vi "DAQ comm.vi"(7 "DAQ T state cluster in":T1={"DAQ state"=enum."Global comm", "device"="Dev1", "start (ms)"=0, "error"={"status"=FALSE, "code"=0, "source"=""}, "T cont"={"exec"={"T mode"=enum."Setting up", "man power"=0.0, "log"=FALSE}, "T status"={"Temp"=0.0, "Power"=0.0}, "utility"={"meas index"=300, "wait (ms)"=0, "H Vmax"=8.5, "power out"=0.0, "heat volt out"=0.0, "heat volt in"=0.0, "therm volt"=0.0, "t T P hist"=[]}}} {"T cont"."utility"."therm volt" format="%_6g"; "T cont"."utility"."heat volt in" format="%_6g"; "T cont"."utility"."heat volt out" format="%_6g"; "T cont"."utility"."power out" format="%_6g"; "T cont"."utility"."H Vmax" format="%_6g"; "T cont"."exec"."man power" format="%_6g"; "T cont"."T status"."Power" format="%_6g"; "T cont"."T status"."Temp" format="%_6g"}) -> (8 "DAQ T state cluster out":T1={"DAQ state"=enum."Global comm", "device"="Dev1", "start (ms)"=0, "error"={"status"=FALSE, "code"=0, "source"=""}, "T cont"={"exec"={"T mode"=enum."Listening to exec", "man power"=0.0, "log"=FALSE}, "T status"={"Temp"=0.0, "Power"=0.0}, "utility"={"meas index"=0, "wait (ms)"=0, "H Vmax"=8.5, "power out"=5.0, "heat volt out"=0.0, "heat volt in"=0.0, "therm volt"=0.0, "t T P hist"=[]}}} {"T cont"."utility"."therm volt" format="%_6g"; "T cont"."utility"."heat volt in" format="%_6g"; "T cont"."utility"."heat volt out" format="%_6g"; "T cont"."utility"."power out" format="%_6g"; "T cont"."utility"."H Vmax" format="%_6g"; "T cont"."exec"."man power" format="%_6g"; "T cont"."T status"."Power" format="%_6g"; "T cont"."T status"."Temp" format="%_6g"})   [LabVIEW 2019]
doc: "This subVI is one of the states of the DAQ state machine in the bug experiment.\n\nThis state monitors the global variables used in the bug experiment. Depending upon the T control mode, it can be transient, or a dwell state with indefinite dwell time while waiting to engage the DAQ interfacing.\n\nPaul K Dixon\nP3600\nCSUSB Physics"
uses:
  typedefs/DAQ T state cluster.ctl
  typedefs/DAQ T state enum.ctl
  typedefs/temp cont cluster.ctl
  typedefs/temp exec cluster.ctl
  typedefs/temp mode enum.ctl
  typedefs/temp indicator.ctl
  typedefs/temp cont utility.ctl
  globals/Bug man temp globals.vi
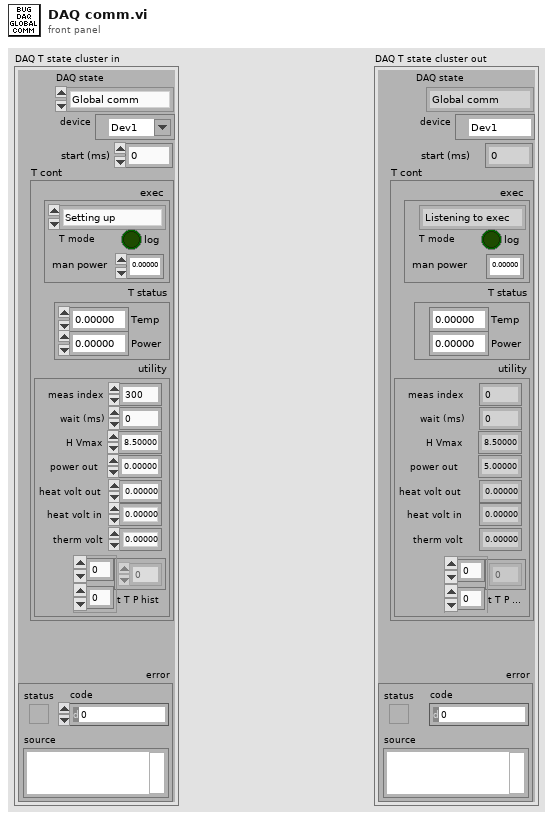
[diagram p1: front panel]
types:
  T1 = typedef "DAQ T state cluster.ctl" = cluster{"DAQ state":T2, "device":tag, "start (ms)":i32, "error":errorcluster, "T cont":T3}
  T2 = typedef "DAQ T state enum.ctl" = enum16{"Global comm", "Meas T & P", "Man Power set", "Output Power", "Wait", "Exit"}
  T3 = typedef "temp cont cluster.ctl" = cluster{"exec":T4, "T status":T6, "utility":T7}
  T4 = typedef "temp exec cluster.ctl" = cluster{"T mode":T5, "man power":dbl, "log":bool}
  T5 = typedef "temp mode enum.ctl" = enum16{"Setting up", "Listening to exec", "Exit"}
  T6 = typedef "temp indicator.ctl" = cluster{"Temp":dbl, "Power":dbl}
  T7 = typedef "temp cont utility.ctl" = cluster{"meas index":i32, "wait (ms)":i32, "H Vmax":dbl, "power out":dbl, "heat volt out":dbl, "heat volt in":dbl, "therm volt":dbl, "t T P hist":dbl[][]}
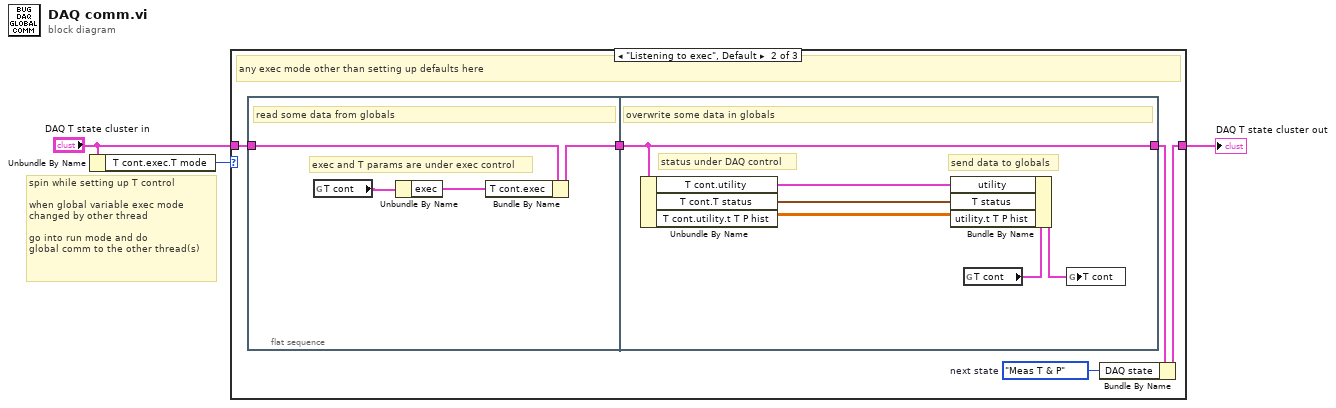
[diagram p0: block diagram]
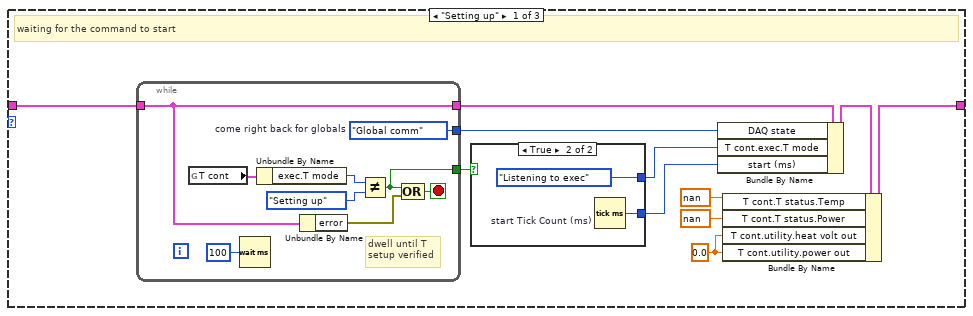
[diagram p2: hidden frame]
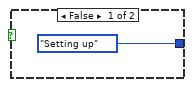
[diagram p3: hidden frame]
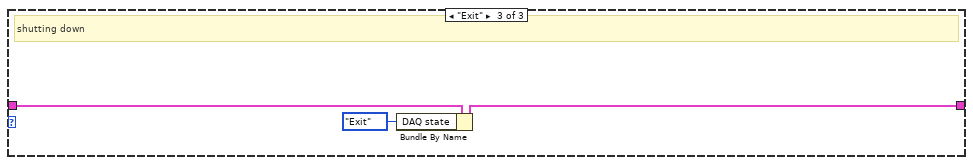
[diagram p4: hidden frame]
diagram:
  # "spin while setting up T control \n\nwhen global variable exec mode\nchanged by other thread\n\ngo into run mode and do\nglobal comm to the other thread(s)"
  n1 = Unbundle By Name("DAQ T state cluster in") -> ("T cont.exec.T mode"=w3:T5)
  n2 = case shown="\"Listening to exec\", Default" w3 {
    tunnel: "DAQ T state cluster in" -> [w14 w31 w44]
    tunnel: [w7 w30 w43] -> w1
    frame "Setting up" {
      w4 = 0.0 ("T cont.heat volt out")
      # "waiting for the command to start"
      n3 = while {
        tunnel: w14 -> [w24]
        tunnel: [w24] -> w13
        tunnel: [w22] -> w12
        tunnel: [w18] -> w10
        stop <- w26 stop-if-true
        w22 = DAQ_T_state_enum."Global comm"  # come right back for globals
        # "dwell until T \nsetup verified"
        n4 = global read "Bug man temp globals.vi" "T cont"() -> (w21:T3)
        n5 = Wait (ms)(milliseconds to wait=u32 100) -> ()  [unwired: 1 out]
        n6 = Unbundle By Name(w21) -> ("exec.T mode"=w20:T5)
        n7 = Unbundle By Name(w24) -> ("error"=w25:errorcluster)
        n8 = Not Equal?(x=w20, y=temp_mode_enum."Setting up" ("exec.T mode")) -> (x != y?=w18:bool)
        n9 = Compound Arithmetic op=OR(w18, w25) -> (w26:bool)
      }
      n10 = case shown="True" w10 {
        tunnel: [temp_mode_enum."Setting up" ("T cont.exec.T mode") temp_mode_enum."Listening to exec" ("T cont.exec.T mode")] -> w11
        tunnel: [_ w16] -> w9
        frame False {
        }
        frame True {
          n11 = Tick Count (ms) "start Tick Count (ms)"() -> (millisecond timer value=w16:u32)
        }
      }
      n12 = Bundle By Name(cluster=w13, "DAQ state"=w12, "T cont.exec.T mode"=w11, "start (ms)"=w9) -> (w8:T1)
      n13 = Bundle By Name(cluster=w8, "T cont.T status.Temp"=nan, "T cont.T status.Power"=nan, "T cont.utility.heat volt out"=w4, "T cont.utility.power out"=w4) -> (w7:T1)
    }
    frame "Listening to exec", Default {
      w29 = DAQ_T_state_enum."Meas T & P"  # next state
      # "any exec mode other than setting up defaults here"
      n14 = flat-sequence {
        tunnel: w31 -> [w35]
        tunnel: [w32] -> w27
        tunnel: [w36] -> w28
        tunnel: w27 -> [w36]
        frame #0 {
          # "exec and T params are under exec control"
          # "read some data from globals"
          n15 = global read "Bug man temp globals.vi" "T cont"() -> (w34:T3)
          n16 = Unbundle By Name(w34) -> ("exec"=w33:T4)
          n17 = Bundle By Name(cluster=w35, "T cont.exec"=w33) -> (w32:T1)
        }
        frame #1 {
          # "status under DAQ control"
          # "send data to globals"
          # "overwrite some data in globals"
          n18 = Unbundle By Name(w36) -> ("T cont.utility"=w37:T7, "T cont.T status"=w39:T6, "T cont.utility.t T P hist"=w38:dbl[][])
          n19 = global read "Bug man temp globals.vi" "T cont"() -> (w41:T3)
          n20 = Bundle By Name(cluster=w41, "utility"=w37, "T status"=w39, "utility.t T P hist"=w38) -> (w40:T3)
          n21 = global write "Bug man temp globals.vi" "T cont"(w40) -> ()
        }
      }
      n22 = Bundle By Name(cluster=w28, "DAQ state"=w29) -> (w30:T1)
    }
    frame "Exit" {
      # "shutting down"
      n23 = Bundle By Name(cluster=w44, "DAQ state"=DAQ_T_state_enum."Exit") -> (w43:T1)
    }
  }
  "DAQ T state cluster out" <- w1
